vi "LCB Get Err Msg.vi"(8 "error in (no error)":errorcluster caption="Fehler (Eingang, kein Fehler)", 11 "Error Code":i32) -> (0 "error out":errorcluster caption="Fehler (Ausgang)", 3 "Error Message":string)   [LabVIEW 2023, in "labbCAN_Bus_API.lvlib"]
doc: "LCB_Func long __stdcall LCB_GetErrMsg(long ErrCode,\n char *pMsgBuf,\n int MsgBufSize);"
uses:
  labbCAN_Bus_API.lvlib
  labbCAN_Bus_API.dll
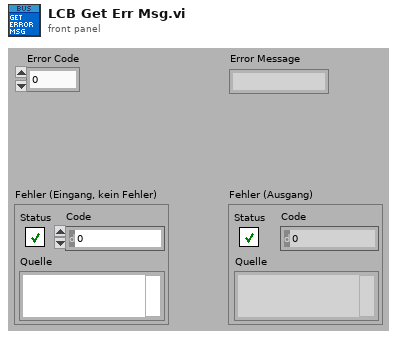
[diagram p1: front panel]
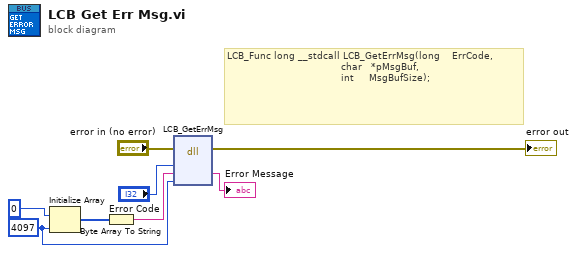
[diagram p0: block diagram]
diagram:
  w1 = 4097 ("Dimension")
  # "LCB_Func long __stdcall LCB_GetErrMsg(long    ErrCode,\n                                      char   *pMsgBuf,\n                                      int     MsgBufSize);"
  n1 = Initialize Array(u8 0 ("Element"), w1) -> (w7:u8[])
  n2 = Byte Array To String(unsigned byte array=w7) -> (string=w6:string)
  n3 = dll-call lib="C:/GIT/DensityGradientProject/CETONI_SDK/labbCAN_Bus_API.*" fn="LCB_GetErrMsg"(error in="error in (no error)", "ErrCode"="Error Code", "pMsgBuf"=w6, "MsgBufSize"=w1) -> (error out=→"error out":errorcluster, "pMsgBuf"=→"Error Message":string)  [unwired: 5 in, 1 out]
